vi "subGetListOfAllFilesToCheck.vi"(11 "Path to Check":path) -> (3 "All Files in Dir":path[](array[path]))   [LabVIEW 2020, in "DependencyInspection.lvlib" / "CDependencyInspection.lvclass"]
uses:
  CDependencyInspection.lvclass
  <vilib>/Utility/LVLibp/NI_PackedLibraryUtility.lvlib
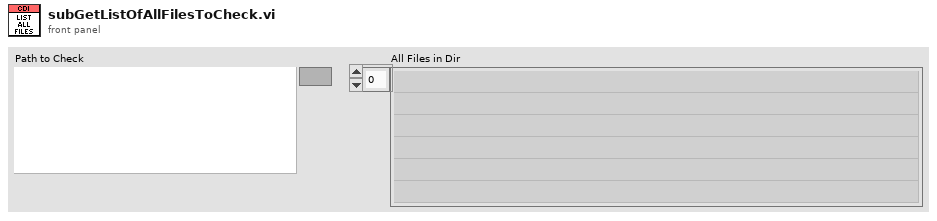
[diagram p1: front panel]
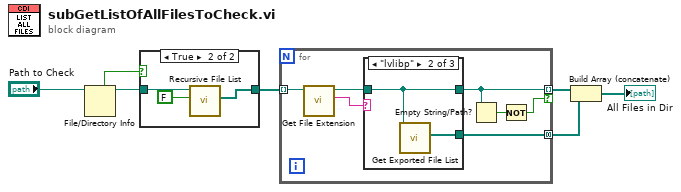
[diagram p0: block diagram]
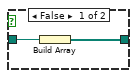
[diagram p2: hidden frame]
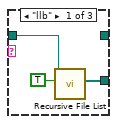
[diagram p3: hidden frame]
diagram:
  n1 = File/Directory Info(path="Path to Check") -> (path out=w6:path, directory=w7:bool)  [unwired: 1 in, 5 out]
  n2 = case shown="True" w7 {
    tunnel: [w9 w10] -> w1
    tunnel: w6 -> [w8 w12]
    frame False {
      n3 = Build Array(w8) -> (w9:path[])
    }
    frame True {
      n4 = call <vilib>:"Recursive File List.vi"("Treat LLBs as Folders?"=FALSE, "Folder Path"=w12) -> ("All Files in Dir"=w10:path[])  [unwired: 5 in, 4 out]
    }
  }
  n5 = for {
    tunnel: w1 -> [w17] mode=indexing
    tunnel: [w16] -> w4 mode=indexing if=w13
    tunnel: [w14] -> w3 mode=concatenating
    n6 = call <vilib>:"Get File Extension.vi"("file"=w17) -> ("lowercase file extension"=w18:string, "dup file"=w19:path)  [unwired: 6 in, 3 out]
    n7 = case shown="\"lvlibp\"" w18 {
      tunnel: w19 -> [w22 w23 w25]
      tunnel: [w21 w24 _] -> w14
      tunnel: [_ w23 w25] -> w16
      frame "llb" {
        n8 = call <vilib>:"Recursive File List.vi"("Treat LLBs as Folders?"=TRUE, "Folder Path"=w22) -> ("All Files in Dir"=w21:path[])  [unwired: 5 in, 4 out]
      }
      frame "lvlibp" {
        n9 = call <vilib>:"Get Exported File List.vi"("packed library path"=w23) -> ("paths"=w24:path[])  [unwired: 8 in, 2 out]
      }
      frame Default {
      }
    }
    n10 = Empty String/Path?(string/path=w16) -> (empty?=w15:bool)
    n11 = Not(x=w15) -> (.not. x?=w13:bool)
  }
  n12 = Build Array (concatenate)(w4, w3) -> (→"All Files in Dir":path[])
